vi "End Bus_Monitor_API StreamBus.vi"(8 "error in":errorcluster, 10 "Cancel All Reads (F)":bool, 11 "Call ID in":T2) -> (0 "error out":errorcluster, 1 "errorDetails":T1)   [LabVIEW 2025, in "bus_monitor_client.lvlib"]
uses:
  bus_monitor_client.lvlib
  <vilib>/gRPC/LabVIEW gRPC Library/Shared/grpcId.ctl
  <vilib>/gRPC/LabVIEW gRPC Library/Shared/Any.ctl
  <vilib>/gRPC/LabVIEW gRPC Library/grpc-lvsupport-release.lvlib
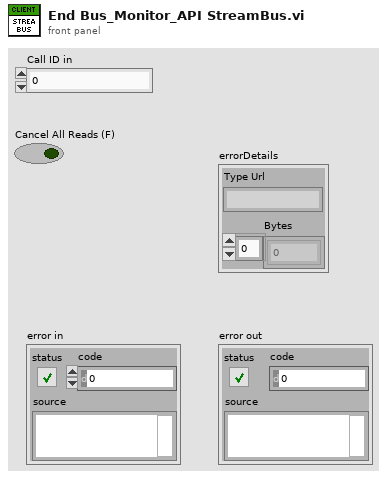
[diagram p1: front panel]
types:
  T1 = typedef "grpc-lvsupport-release.lvlib/Any.ctl" = cluster{"Type Url":string, "Bytes":u8[]}
  T2 = typedef "grpc-lvsupport-release.lvlib/grpcId.ctl" = u64
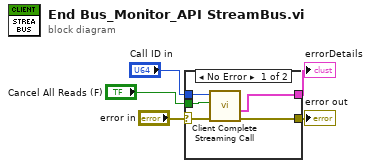
[diagram p0: block diagram]
diagram:
  n1 = case shown="No Error" "error in" {
    selector: "error in" -> [w10 w11]
    tunnel: [w9 w11] -> w4
    tunnel: "Call ID in" -> [w8 _]
    tunnel: [w7 _] -> w2
    tunnel: "Cancel All Reads (F)" -> [w6 _]
    frame No Error {
      n2 = call <vilib>:"Client Complete Streaming Call.vi"("error in"=w10, "Cancel All Reads (F)"=w6, "Call ID in"=w8) -> ("error out"=w9:errorcluster, "errorDetails"=w7:T1)  [unwired: 7 in]
    }
    frame Error {
    }
  }
  "error out" <- w4
  "errorDetails" <- w2
